vi "Move Files.vi"(8 "error in (no error)":errorcluster, 9 "Enable":bool=TRUE, 10 "Target Directory":path=path "D:/Data", 11 "Files to Move":path[](array[path])) -> (0 "error out":errorcluster)   [LabVIEW 2009]
panel:
  out "standard output":string
  out "concatenated string":string
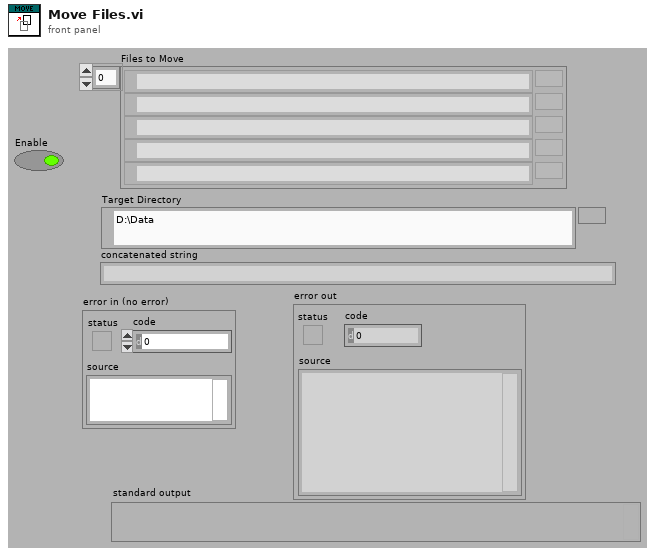
[diagram p1: front panel]
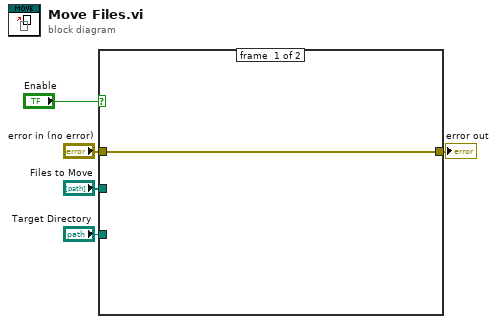
[diagram p0: block diagram]
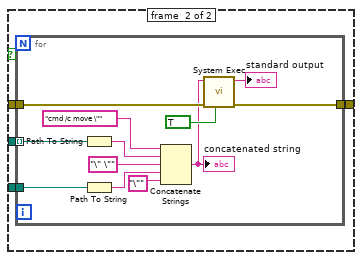
[diagram p2: hidden frame]
diagram:
  n1 = case shown="True" "Enable" {
    tunnel: "Files to Move" -> [_ w10]
    tunnel: "Target Directory" -> [_ w9]
    tunnel: "error in (no error)" -> [w6 w8]
    tunnel: [w6 w7] -> w2
    frame #0 {
    }
    frame #1 {
      n2 = for {
        tunnel: w10 -> [w22] mode=indexing
        tunnel: w9 -> [w18]
        tunnel: w8 -> [w15]
        tunnel: [w14] -> w7
        n3 = Path To String(path=w22) -> (string=w20:string)
        n4 = Path To String(path=w18) -> (string=w17:string)
        n5 = Concatenate Strings("cmd /c move \"", w20, "\" \"" ("string"), w17, "\"" ("string")) -> (w12:string)
        "concatenated string" <- w12
        n6 = call <vilib>:"System Exec.vi"("run minimized? (F)"=TRUE, "error in (no error)"=w15, "command line"=w12) -> ("error out"=w14:errorcluster, "standard output"=→"standard output":string)  [unwired: 5 in, 2 out]
      }
    }
  }
  "error out" <- w2
